vi "PuertaGarageConPausas.vi"() -> ()   [LabVIEW 2018]
panel:
  in  "stop":bool
  out "Slide":i8(slide)=6 scale=0.0..6.0
  out "H0":bool
  out "H1":bool
  in  "Persona":bool
  in  "S":bool
  in  "Down":bool
  in  "Up":bool
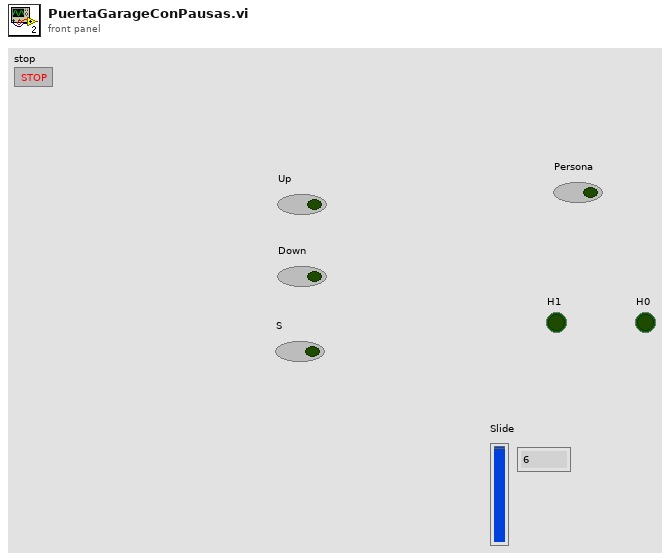
[diagram p1: front panel]
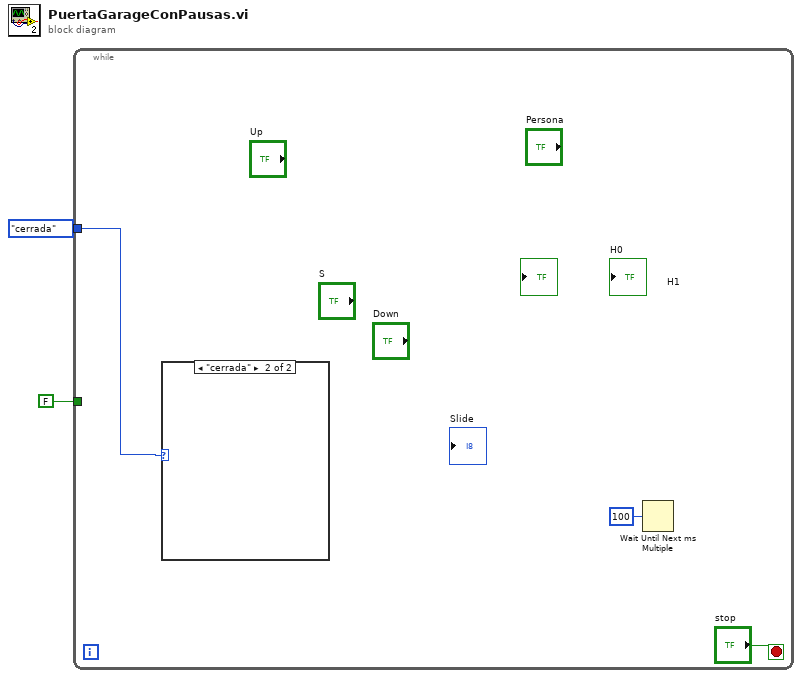
[diagram p0: block diagram]
diagram:
  n1 = while {
    tunnel: enum16{"cerrada"}."cerrada" -> [w3]
    tunnel: FALSE -> [_]
    stop <- "stop" stop-if-true
    n2 = case shown="\"1\"" w3 {
      frame "cerrada", Default {
      }
      frame "cerrada" {
      }
    }
    n3 = Wait Until Next ms Multiple(millisecond multiple=u32 100) -> ()  [unwired: 1 out]
  }
